vi "validarteChecksum.vi"(6 "messageType":T1, 8 "error in (no error)":errorcluster, 9 "checkSum":string, 10 "response":string, 11 "CoolerSerialCommand in":refnum<class "CoolerSerialCommand.lvclass">) -> (0 "error out":errorcluster, 2 "validChecksum":bool, 3 "CoolerSerialCommand out":refnum<class "CoolerSerialCommand.lvclass">)   [LabVIEW 2016, in "CoolerSerialCommand.lvclass"]
uses:
  CoolerSerialCommand.lvclass
  typedefs/typeOfCommand.ctl
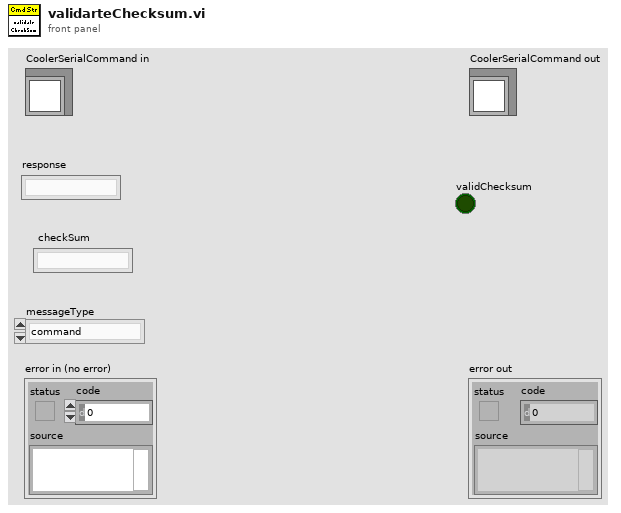
[diagram p1: front panel]
types:
  T1 = typedef "typeOfCommand.ctl" = enum16{"command", "response"}
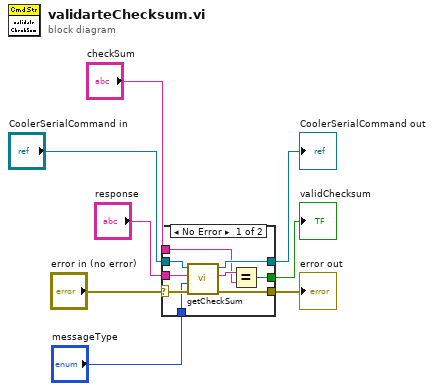
[diagram p0: block diagram]
diagram:
  n1 = case shown="No Error" "error in (no error)" {
    selector: "error in (no error)" -> [w15 w19]
    tunnel: [w14 w19] -> w7
    tunnel: [w16 w18] -> w5
    tunnel: "CoolerSerialCommand in" -> [w17 w18]
    tunnel: "response" -> [w13 _]
    tunnel: "checkSum" -> [w11 _]
    tunnel: [w10 _] -> w2
    tunnel: "messageType" -> [w9 _]
    frame No Error {
      n2 = call "getCheckSum.vi"("error in (no error)"=w15, "messageType"=w9, "response"=w13, "CoolerSerialCommand in"=w17) -> ("error out"=w14:errorcluster, "Checksum"=w12:string, "CoolerSerialCommand out"=w16:refnum<class "CoolerSerialCommand.lvclass">)  [unwired: 5 in]
      n3 = Equal?(x=w12, y=w11) -> (x = y?=w10:bool)
    }
    frame Error {
    }
  }
  "error out" <- w7
  "CoolerSerialCommand out" <- w5
  "validChecksum" <- w2
